vi "cage rotator.vi"(5 "Action":T4, 7 "Set/Get":T3=enum."Get", 8 "Error In":errorcluster, 9 "Cage rotator":T1={"Position"=0.0, "Is.Enabled?"=FALSE, "Is.Connected?"=FALSE, "Device SN"="55151324", "AccelerationMaximum"=10.0, "VelocityMaximum"=10.0, "Acceleration"=10.0, "Velocity"=10.0, "waitTimeout (ms)"=100000, "Model"=enum."None", "Is.Homed?"=FALSE}) -> (0 "Error Out":errorcluster, 1 "Cluster Out":T1={"Position"=0.0, "Is.Enabled?"=FALSE, "Is.Connected?"=FALSE, "Device SN"="45876539", "AccelerationMaximum"=0.0, "VelocityMaximum"=0.0, "Acceleration"=0.0, "Velocity"=0.0, "waitTimeout (ms)"=0, "Model"=enum."None", "Is.Homed?"=FALSE})   [LabVIEW 2018]
uses:
  Thorlabs Translation Stages/Controls/Motion Translation Module Control.ctl
  General/Controls/Set Get Controls.ctl
  Thorlabs Translation Stages/Controls/Translation Stage Cluster.ctl
  General/Controls/Translation Stage Types.ctl
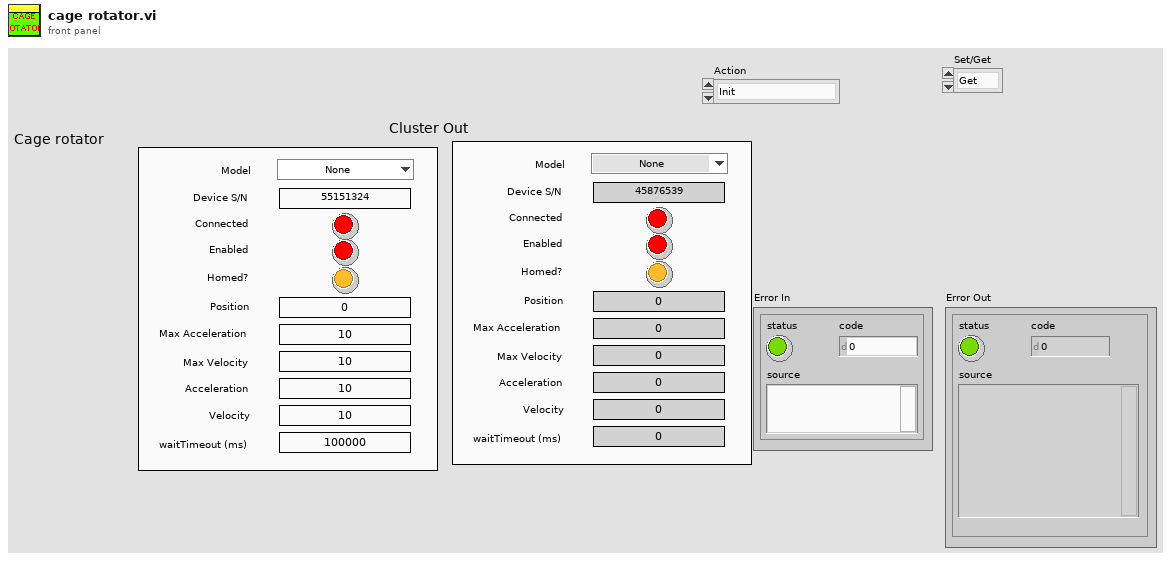
[diagram p1: front panel]
types:
  T1 = typedef "Translation Stage Cluster.ctl" = cluster{"Position":dbl, "Is.Enabled?":bool, "Is.Connected?":bool, "Device SN":string, "AccelerationMaximum":dbl, "VelocityMaximum":dbl, "Acceleration":dbl, "Velocity":dbl, "waitTimeout (ms)":i32, "Model":T2, "Is.Homed?":bool}
  T2 = typedef "Translation Stage Types.ctl" = enum16{"None", "Thorlabs LTS", "Thorlabs MLJ"}
  T3 = typedef "Set Get Controls.ctl" = enum16{"Set", "Get"}
  T4 = typedef "Motion Translation Module Control.ctl" = enum16{"Init", "Home", "Status", "Velocity/Accel", "Position", "Jog", "Stop", "Uninit", "Enable", "Disable"}
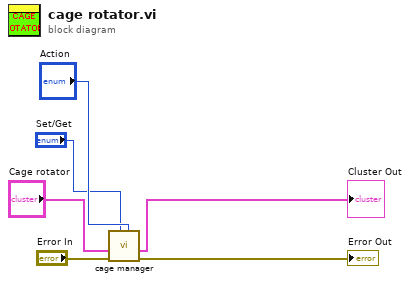
[diagram p0: block diagram]
diagram:
  n1 = call "cage manager.vi"("Action"="Action", "Set/Get"="Set/Get", "Error In"="Error In", "Cluster In"="Cage rotator") -> ("Error Out"=→"Error Out":errorcluster, "Cluster Out"=→"Cluster Out":T1)  [unwired: 6 in]
